vi "Init Ring Picture.vi"(8 "error in (no error)":errorcluster, 11 "[V] Login in":refnum<class "[V] Login.lvclass">) -> (0 "error out":errorcluster, 3 "[V] Login out":refnum<class "[V] Login.lvclass">)   [LabVIEW 2020, in "[V] Login.lvlib" / "[V] Login.lvclass"]
uses:
  [V] Login.lvclass
  [V] Login.lvclass/[V] Login.ctl
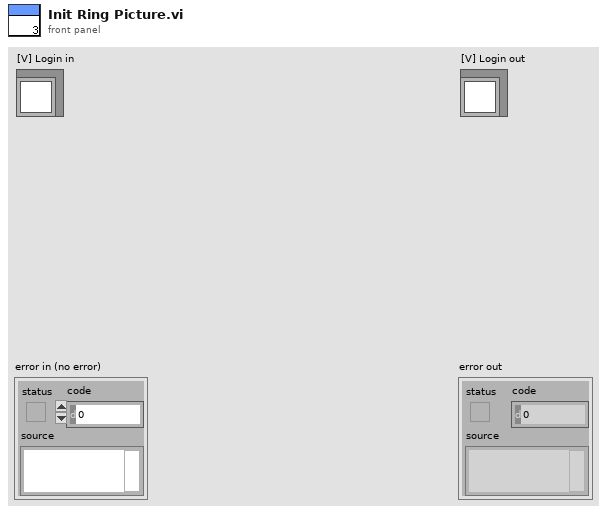
[diagram p1: front panel]
types:
  T1 = typedef "imagedata.ctl" = cluster{"image type":i32, "image depth":i32, "image":u8[], "mask":u8[], "colors":u32[], "Rectangle":cluster{"left":i16, "top":i16, "right":i16, "bottom":i16}}
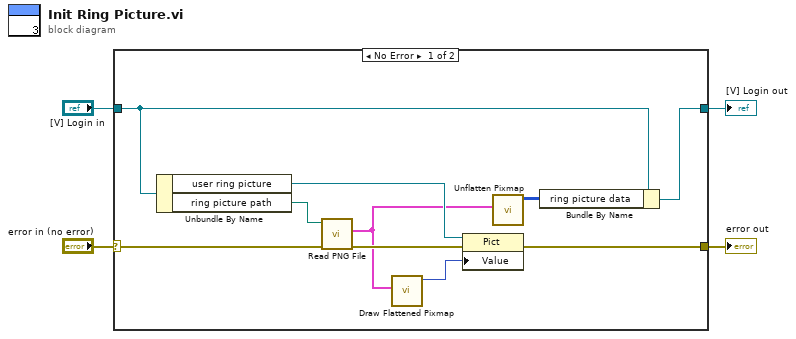
[diagram p0: block diagram]
diagram:
  n1 = case shown="No Error" "error in (no error)" {
    selector: "error in (no error)" -> [w14 w16]
    tunnel: [w5 w16] -> w3
    tunnel: [w6 w15] -> w1
    tunnel: "[V] Login in" -> [w8 w15]
    frame No Error {
      n2 = Unbundle By Name(w8) -> ("user ring picture"=w11:refnum<vi>, "ring picture path"=w13:path)
      n3 = call <vilib>:"Read PNG File.vi"("error in (no error)"=w14, "path to PNG file"=w13) -> ("error out"=w12:errorcluster, "image data"=w9:T1)  [unwired: 7 in, 1 out]
      n4 = call <vilib>:"Draw Flattened Pixmap.vi"("image data"=w9) -> ("new picture"=w10:picture)  [unwired: 8 in]
      n5 = property class="Pict"(reference=w11, error in=w12, "Value"=w10) -> (error out=w5:errorcluster)  [unwired: 1 out]
      n6 = call <vilib>:"Unflatten Pixmap.vi"("image data"=w9) -> ("24-bit pixmap"=w7:u32[][])  [unwired: 4 in, 6 out]
      n7 = Bundle By Name(cluster=w8, "ring picture data"=w7) -> (w6:refnum<class "[V] Login.lvclass">)
    }
    frame Error {
    }
  }
  "error out" <- w3
  "[V] Login out" <- w1
